vi "ArmDontScrapeCargoHoop.vi"(2 "InputPath":T2[](array[typedef]), 3 "RobotDimensions":T1) -> (0 "OutputPath":T2[](array[typedef]))   [LabVIEW 2018]
uses:
  TypeDefs/ArmAbsolutePosition.ctl
  TypeDefs/ConfigComponents/Config_Dimensions.ctl
panel:
  in  "VerticalBuffer (in)":dbl=3.0
  in  "VerticalTolerance (rad)":dbl=0.25
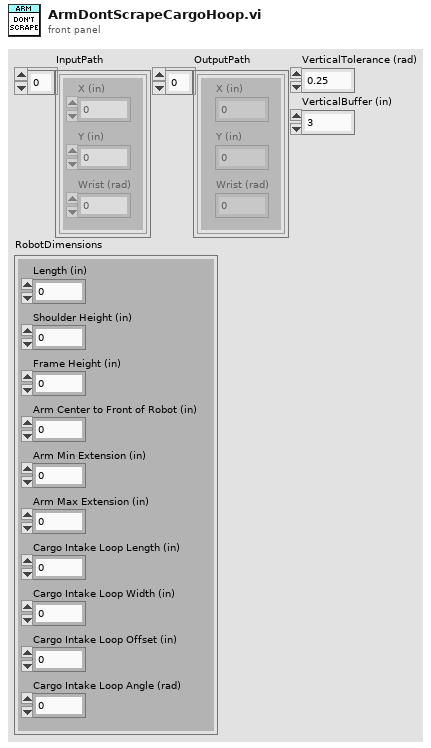
[diagram p1: front panel]
types:
  T1 = typedef "Config_Dimensions.ctl" = cluster{"Length (in)":dbl, "Shoulder Height (in)":dbl, "Frame Height (in)":dbl, "Arm Center to Front of Robot (in)":dbl, "Arm Min Extension (in)":dbl, "Arm Max Extension (in)":dbl, "Cargo Intake Loop Length (in)":dbl, "Cargo Intake Loop Width (in)":dbl, "Cargo Intake Loop Offset (in)":dbl, "Cargo Intake Loop Angle (rad)":dbl}
  T2 = typedef "ArmAbsolutePosition.ctl" = cluster{"X (in)":dbl, "Y (in)":dbl, "Wrist (rad)":dbl}
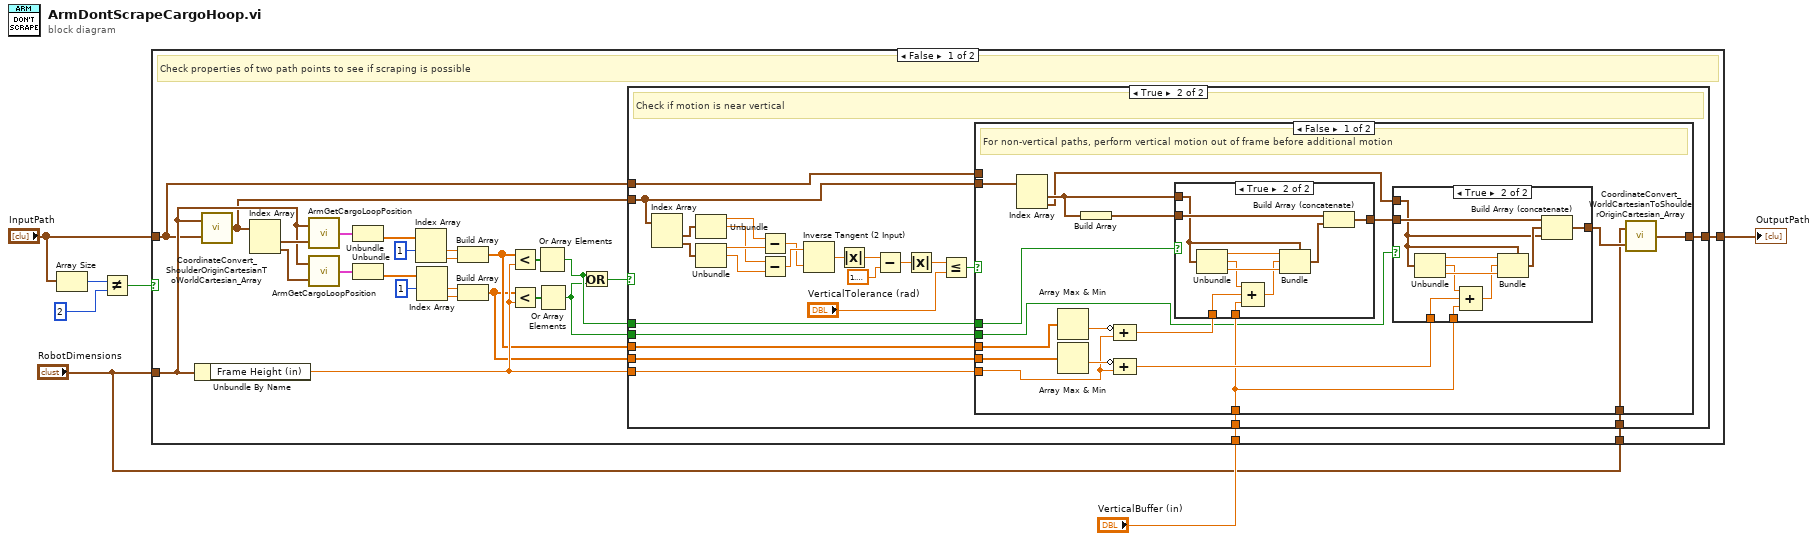
[diagram p0: block diagram]
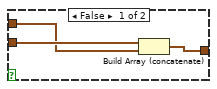
[diagram p3: hidden frame]
diagram:
  n1 = Array Size(array="InputPath") -> (size(s)=w7:i32)
  n2 = Not Equal?(x=w7, y=2) -> (x != y?=w5:bool)
  n3 = case shown="False" w5 {
    tunnel: [w16 w103] -> w3
    tunnel: "InputPath" -> [w17 w103]
    tunnel: "RobotDimensions" -> [w31 _]
    tunnel: "VerticalBuffer (in)" -> [w9 _]
    tunnel: "RobotDimensions" -> [w8 _]
    frame False {
      # "Check properties of two path points to see if scraping is possible"
      n4 = Unbundle By Name(w31) -> ("Frame Height (in)"=w14:dbl)
      n5 = call "CoordinateConvert_ShoulderOriginCartesianToWorldCartesian_Array.vi"("ArmPositionRelativeToShoulderIn"=w17, "RobotDimensions"=w31) -> ("ArmAbsolutePosition"=w15:T2[])
      n6 = Index Array(array=w15) -> (element #1=w33:T2, element #2=w32:T2)  [unwired: 2 in]
      n7 = call "ArmGetCargoLoopPosition.vi"("ArmAbsolutePose"=w33, "RobotDimensions"=w31) -> ("CargoLoopPoints"=w30:cluster{dbl[], dbl[]})
      n8 = call "ArmGetCargoLoopPosition.vi"("ArmAbsolutePose"=w32, "RobotDimensions"=w31) -> ("CargoLoopPoints"=w29:cluster{dbl[], dbl[]})
      n9 = Unbundle(w30) -> (w25:dbl[])  [unwired: 1 out]
      n10 = Unbundle(w29) -> (w28:dbl[])  [unwired: 1 out]
      n11 = Index Array(array=w25, index #1=1 ("index")) -> (element #1=w24:dbl, element #2=w23:dbl)  [unwired: 1 in]
      n12 = Index Array(array=w28, index #1=1 ("index")) -> (element #1=w21:dbl, element #2=w22:dbl)  [unwired: 1 in]
      n13 = Build Array(w24, w23) -> (w11:dbl[])
      n14 = Build Array(w21, w22) -> (w10:dbl[])
      n15 = Less?(x=w11, y=w14) -> (x < y?=w19:bool[])
      n16 = Less?(x=w10, y=w14) -> (x < y?=w20:bool[])
      n17 = Or Array Elements(Boolean array=w19) -> (logical OR=w13:bool)
      n18 = Or Array Elements(Boolean array=w20) -> (logical OR=w12:bool)
      n19 = Or(x=w13, y=w12) -> (x .or. y?=w18:bool)
      n20 = case shown="True" w18 {
        tunnel: w17 -> [w34 w44]
        tunnel: [w34 w43] -> w16
        tunnel: w15 -> [_ w42]
        tunnel: w14 -> [_ w41]
        tunnel: w13 -> [_ w40]
        tunnel: w12 -> [_ w39]
        tunnel: w11 -> [_ w38]
        tunnel: w10 -> [_ w37]
        tunnel: w9 -> [_ w36]
        tunnel: w8 -> [_ w35]
        frame False {
          # "Endpoints are above the frame"
        }
        frame True {
          # "Check if motion is near vertical"
          n21 = Index Array(array=w42) -> (element #1=w59:T2, element #2=w58:T2)  [unwired: 2 in]
          n22 = Unbundle(w59) -> ("X (in)"=w57:dbl, "Y (in)"=w55:dbl)  [unwired: 1 out]
          n23 = Unbundle(w58) -> ("X (in)"=w56:dbl, "Y (in)"=w54:dbl)  [unwired: 1 out]
          n24 = Subtract(x=w57, y=w56) -> (x-y=w52:dbl)
          n25 = Subtract(x=w55, y=w54) -> (x-y=w53:dbl)
          n26 = Inverse Tangent (2 Input)(1:w52, 2:w53) -> (0:w51:dbl)
          n27 = Absolute Value(x=w51) -> (abs(x)=w50:dbl)
          n28 = Subtract(x=w50, y=1.5707963267948966) -> (x-y=w48:dbl)
          n29 = Absolute Value(x=w48) -> (abs(x)=w47:dbl)
          n30 = Less Or Equal?(x=w47, y="VerticalTolerance (rad)") -> (x <= y?=w45:bool)
          n31 = case shown="False" w45 {
            tunnel: w44 -> [_ w102]
            tunnel: [w61 w102] -> w43
            tunnel: w42 -> [w71 _]
            tunnel: w41 -> [w73 _]
            tunnel: w40 -> [w72 _]
            tunnel: w39 -> [w63 _]
            tunnel: w38 -> [w77 _]
            tunnel: w37 -> [w76 _]
            tunnel: w36 -> [w64 _]
            tunnel: w35 -> [w60 _]
            frame False {
              # "For non-vertical paths, perform vertical motion out of frame before additional motion"
              n32 = Index Array(array=w71) -> (element #1=w69:T2, element #2=w66:T2)  [unwired: 2 in]
              n33 = Array Max & Min(array=w77) -> (min value=w74:dbl)  [unwired: 3 out]
              n34 = Array Max & Min(array=w76) -> (min value=w75:dbl)  [unwired: 3 out]
              n35 = Build Array(w69) -> (w70:T2[])
              n36 = Compound Arithmetic op=ADD(invert w74, w73) -> (w68:dbl)
              n37 = Compound Arithmetic op=ADD(invert w75, w73) -> (w65:dbl)
              n38 = case shown="True" w72 {
                tunnel: w70 -> [w91 w101]
                tunnel: w69 -> [_ w100]
                tunnel: [w91 w97] -> w67
                tunnel: w68 -> [_ w94]
                tunnel: w64 -> [_ w93]
                frame False {
                }
                frame True {
                  n39 = Unbundle(w100) -> ("X (in)"=w99:dbl, "Y (in)"=w95:dbl, "Wrist (rad)"=w98:dbl)
                  n40 = Compound Arithmetic op=ADD(w95, w94, w93) -> (w92:dbl)
                  n41 = Bundle(cluster=w100, "X (in)"=w99, "Y (in)"=w92, "Wrist (rad)"=w98) -> (w96:T2)
                  n42 = Build Array (concatenate)(w101, w96) -> (w97:T2[])
                }
              }
              n43 = case shown="True" w63 {
                tunnel: w67 -> [w80 w83]
                tunnel: w66 -> [w79 w81]
                tunnel: [w78 w88] -> w62
                tunnel: w65 -> [_ w86]
                tunnel: w64 -> [_ w85]
                frame False {
                  n44 = Build Array (concatenate)(w80, w79) -> (w78:T2[])
                }
                frame True {
                  n45 = Unbundle(w81) -> ("X (in)"=w90:dbl, "Y (in)"=w87:dbl, "Wrist (rad)"=w89:dbl)
                  n46 = Compound Arithmetic op=ADD(w87, w86, w85) -> (w84:dbl)
                  n47 = Bundle(cluster=w81, "X (in)"=w90, "Y (in)"=w84, "Wrist (rad)"=w89) -> (w82:T2)
                  n48 = Build Array (concatenate)(w83, w82, w81) -> (w88:T2[])
                }
              }
              n49 = call "CoordinateConvert_WorldCartesianToShoulderOriginCartesian_Array.vi"("ArmPositionIn"=w62, "RobotDimensions"=w60) -> ("ArmPositionRelativeToShoulder"=w61:T2[])
            }
            frame True {
              # "Allow vertical motion"
            }
          }
        }
      }
    }
    frame True {
      # "Either no points or the wrong number of points for checking"
    }
  }
  "OutputPath" <- w3
